vi "ParseServerData.vi"(6 "通道选择ref":refnum<vi>[](array[refnum]), 8 "error in (no error)":errorcluster, 9 "试验箱选择":refnum<vi>, 10 "This VI":refnum<vi>, 11 "ServerData":T4) -> (0 "error out":errorcluster, 3 "SelectedDeviceChannelsData":T1[](array[typedef]))   [LabVIEW 2010]
uses:
  Ctrls/ServerData.ctl
  Ctrls/DeviceInfomation.ctl
  Ctrls/DeviceModel.ctl
  Ctrls/ChannelData.ctl
  Ctrls/ChannelType.ctl
  Ctrls/ChannelAccessType.ctl
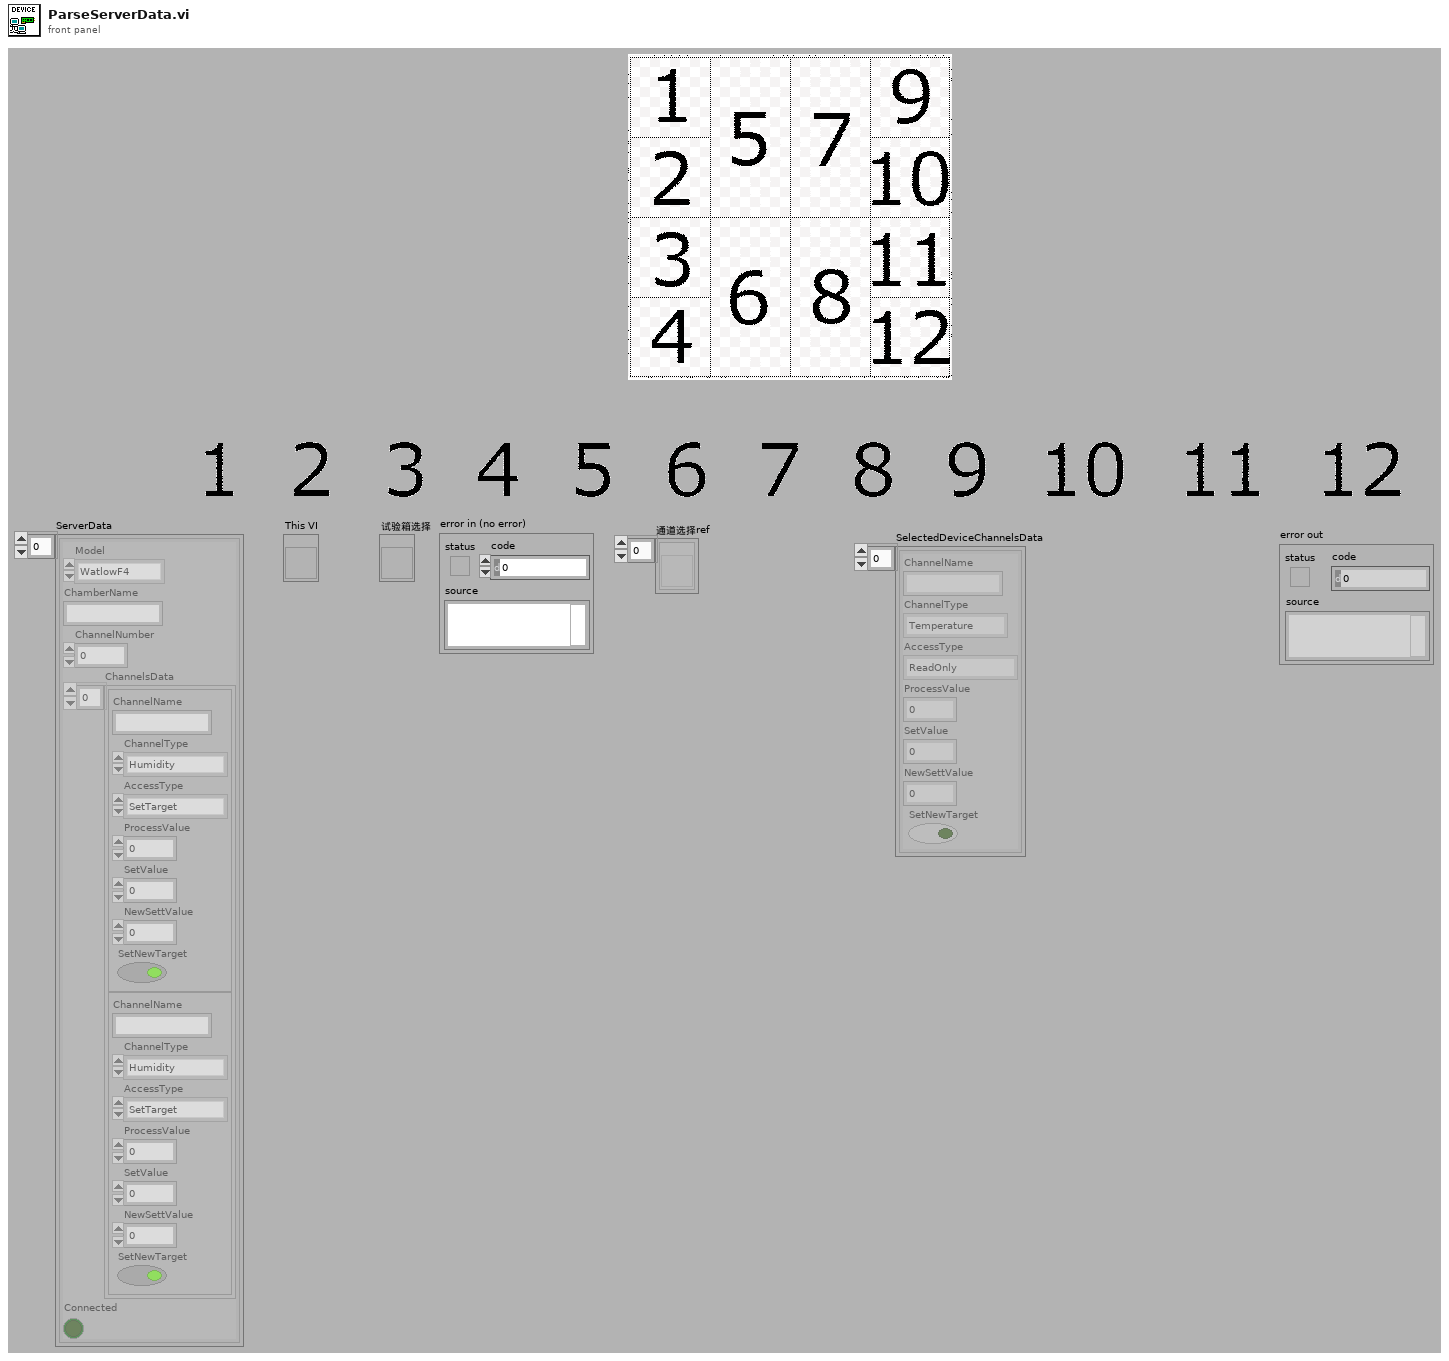
[diagram p1: front panel]
types:
  T1 = typedef "ChannelData.ctl" = cluster{"ChannelName":string, "ChannelType":T2, "AccessType":T3, "ProcessValue":dbl, "SetValue":dbl, "NewSettValue":dbl, "SetNewTarget":bool}
  T2 = typedef "ChannelType.ctl" = enum16{"Temperature", "Humidity"}
  T3 = typedef "ChannelAccessType.ctl" = enum16{"ReadOnly", "SetTarget"}
  T4 = typedef "ServerData.ctl" = T5[]
  T5 = typedef "DeviceInfomation.ctl" = cluster{"Model":T6, "ChamberName":string, "ChannelNumber":i32, "ChannelsData":T1[], "Connected":bool}
  T6 = typedef "DeviceModel.ctl" = enum16{"WatlowF4", "CenterOne", "DCP551", "DPR250"}
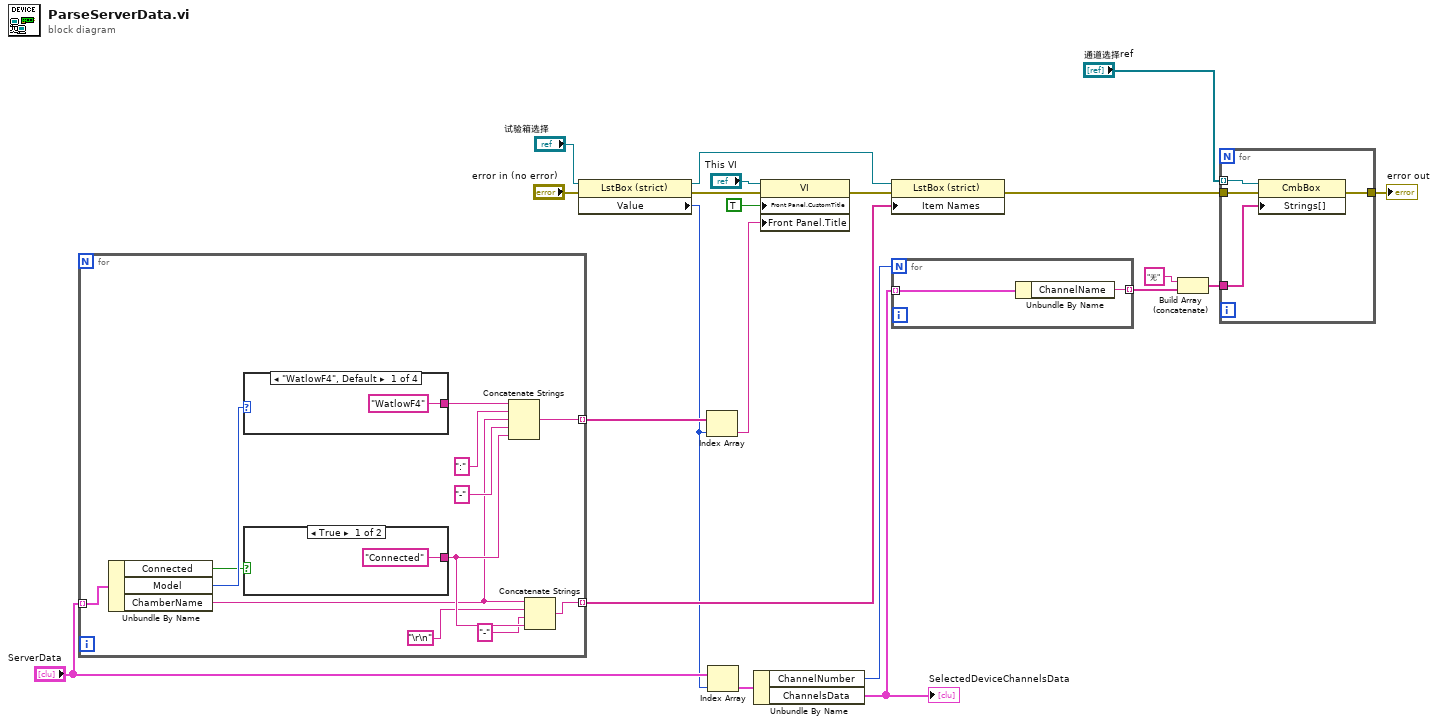
[diagram p0: block diagram]
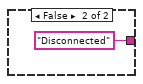
[diagram p2: hidden frame]
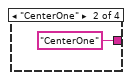
[diagram p3: hidden frame]
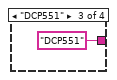
[diagram p4: hidden frame]
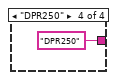
[diagram p5: hidden frame]
diagram:
  n1 = for {
    tunnel: "ServerData" -> [w33] mode=indexing
    tunnel: [w24] -> w17 mode=indexing
    tunnel: [w27] -> w16 mode=indexing
    n2 = Unbundle By Name(w33) -> ("Connected"=w28:bool, "Model"=w32:T6, "ChamberName"=w25:string)
    n3 = case shown="\"WatlowF4\", Default" w32 {
      tunnel: ["WatlowF4" "CenterOne" "DCP551" "DPR250"] -> w31
      frame "WatlowF4", Default {
      }
      frame "CenterOne" {
      }
      frame "DCP551" {
      }
      frame "DPR250" {
      }
    }
    n4 = case shown="True" w28 {
      tunnel: ["Connected" "Disconnected"] -> w26
      frame True {
      }
      frame False {
      }
    }
    n5 = Concatenate Strings(w31, ":" ("string"), w25, "-" ("string"), w26) -> (w27:string)
    n6 = Concatenate Strings(w25, "\r\n", "-" ("string"), w26) -> (w24:string)
  }
  n7 = property class="LstBox (strict)"(reference="试验箱选择", error in="error in (no error)") -> (reference out=w18:refnum<vi>, error out=w14:errorcluster, "Value"=w8:i32)
  n8 = Index Array(array=w16, index=w8) -> (element=w15:string)
  n9 = Index Array(array="ServerData", index=w8) -> (element=w7:T5)
  n10 = Unbundle By Name(w7) -> ("ChannelNumber"=w10:i32, "ChannelsData"=w11:T1[])
  "SelectedDeviceChannelsData" <- w11
  n11 = property class="VI"(reference="This VI", error in=w14, "Front Panel.CustomTitle"=TRUE ("Front Panel Window:Custom Title"), "Front Panel.Title"=w15) -> (error out=w13:errorcluster)  [unwired: 1 out]
  n12 = property class="LstBox (strict)"(reference=w18, error in=w13, "Item Names"=w17) -> (error out=w3:errorcluster)  [unwired: 1 out]
  n13 = for {
    N: w10 -> [_]
    tunnel: w11 -> [w41] mode=indexing
    tunnel: [w40] -> w6 mode=indexing
    n14 = Unbundle By Name(w41) -> ("ChannelName"=w40:string)
  }
  n15 = Build Array (concatenate)("无" ("ChannelName"), w6) -> (w4:string[])
  n16 = for {
    tunnel: "通道选择ref" -> [w45] mode=indexing
    tunnel: w4 -> [w44]
    tunnel: w3 -> [w43]
    tunnel: [w42] -> w2
    n17 = property class="CmbBox"(reference=w45, error in=w43, "Strings[]"=w44) -> (error out=w42:errorcluster)  [unwired: 1 out]
  }
  "error out" <- w2
